vi "parseStatus.vi"(8 "error in (no error)":errorcluster, 9 "timeout":bool=TRUE, 10 "Message":string, 11 "domeCommunicator in":refnum<class "DomeCommunicator.lvclass">) -> (0 "error out":errorcluster, 2 "status":T1, 3 "domeCommunicator out":refnum<class "DomeCommunicator.lvclass">)   [LabVIEW 2016, in "DomeCommunicator.lvclass"]
uses:
  DomeCommunicator.lvclass
  common_labview_tcpdevice/typedefs/deviceStatus.ctl
  common_labview_tcpdevice/typedefs/statusEnum.ctl
  common_labview_tcpdevice/tcpDevice/tcpDevice.lvclass
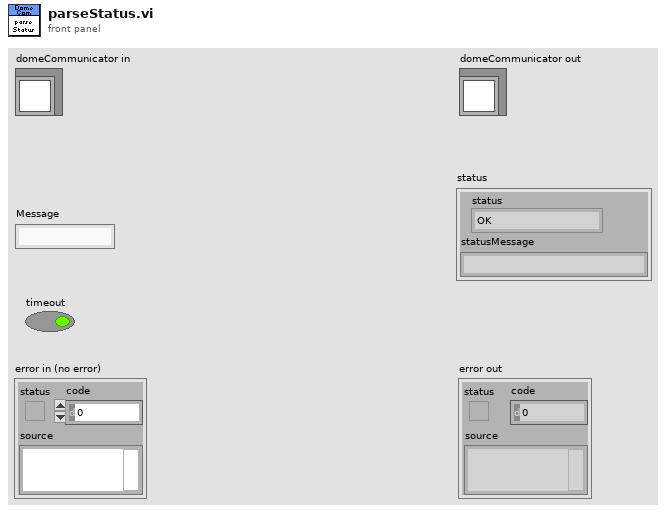
[diagram p1: front panel]
types:
  T1 = typedef "deviceStatus.ctl" = cluster{"status":T2, "statusMessage":string}
  T2 = typedef "statusEnum.ctl" = enum16{"OK", "TIMEOUT", "MSGERROR"}
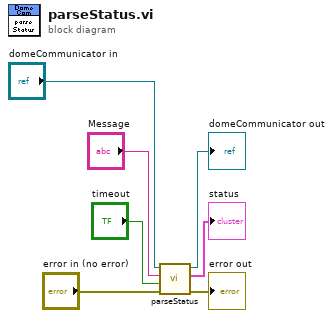
[diagram p0: block diagram]
diagram:
  n1 = call-parent "parseStatus.vi"("error in (no error)"="error in (no error)", "timeout"="timeout", "Message"="Message", "tcpDevice in"="domeCommunicator in") -> ("error out"=→"error out":errorcluster, "status"=→"status":T1, "tcpDevice out"=→"domeCommunicator out":refnum<class "DomeCommunicator.lvclass">)  [unwired: 5 in]
